vi "CHECK SERVER CONECTION.vi"(8 "error in (no error)":errorcluster, 11 "semaphore":T1) -> (0 "error out":errorcluster, 3 "semaphore out":T1)   [LabVIEW 2015]
uses:
  <vilib>/addons/JSON API/JSON Object/Set Object Item by name.vi
  <vilib>/addons/JSON API/JSON Value/Get as JSON string (pretty).vi
  <vilib>/addons/JSON API/JSON Scalar/Set String.vi
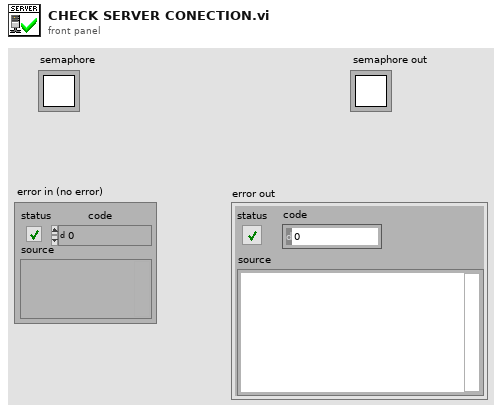
[diagram p1: front panel]
types:
  T1 = typedef "Semaphore RefNum" = refnum<k1>
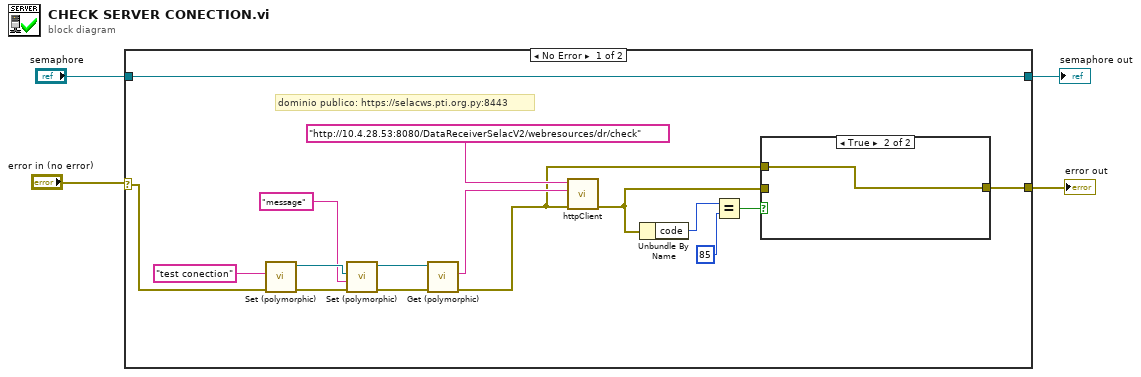
[diagram p0: block diagram]
diagram:
  n1 = case shown="No Error" "error in (no error)" {
    selector: "error in (no error)" -> [w13 w24]
    tunnel: [w9 w24] -> w4
    tunnel: [w11 w23] -> w2
    tunnel: "semaphore" -> [w11 w23]
    frame No Error {
      # "dominio publico: https://selacws.pti.org.py:8443"
      n2 = call-poly <vilib>:"Set (polymorphic).vi"("error in (no error)"=w13, "String"="test conection") -> ("error out"=w15:errorcluster, "JSON Scalar out"=w18:refnum<class "JSON Scalar.lvclass">)  [unwired: 8 in]
      n3 = call-poly <vilib>:"Set (polymorphic).vi"("error in (no error)"=w15, "name"="message", "Value"=w18) -> ("error out"=w14:errorcluster, "JSON Object out"=w16:refnum<class "JSON Object.lvclass">)  [unwired: 6 in, 1 out]
      n4 = call-poly <vilib>:"Get (polymorphic).vi"("error in (no error)"=w14, "JSON Value in"=w16) -> ("error out"=w8:errorcluster, "String"=w12:string)  [unwired: 8 in]
      n5 = call "httpClient.vi"("error in"=w8, "data"=w12, "URI"="http://10.4.28.53:8080/DataReceiverSelacV2/webresources/dr/check") -> ("error out"=w10:errorcluster)  [unwired: 6 in, 2 out]
      n6 = Unbundle By Name(w10) -> ("code"=w6:i32)
      n7 = Equal?(x=w6, y=85) -> (x = y?=w7:bool)
      n8 = case shown="True" w7 {
        tunnel: [w21 w22] -> w9
        tunnel: w10 -> [w21 _]
        tunnel: w8 -> [_ w22]
        frame False {
        }
        frame True {
        }
      }
    }
    frame Error {
    }
  }
  "error out" <- w4
  "semaphore out" <- w2
